vi "Save Image.vi"(8 "error in (no error)":errorcluster, 11 "Save Image in":refnum<class "Save Image.lvclass">) -> (0 "error out":errorcluster, 3 "Save Image out":refnum<class "Save Image.lvclass">)   [LabVIEW 2018, in "Save Image.lvclass"]
uses:
  Save Image.lvclass
  <userlib>/gfitsio/cfitsio-bitpix.ctl
  Save Image.lvclass/Save Image.ctl
  <userlib>/gfitsio/gfitsio-write-image-subset-variant.vi
  <userlib>/gfitsio/gfitsio.lvlib
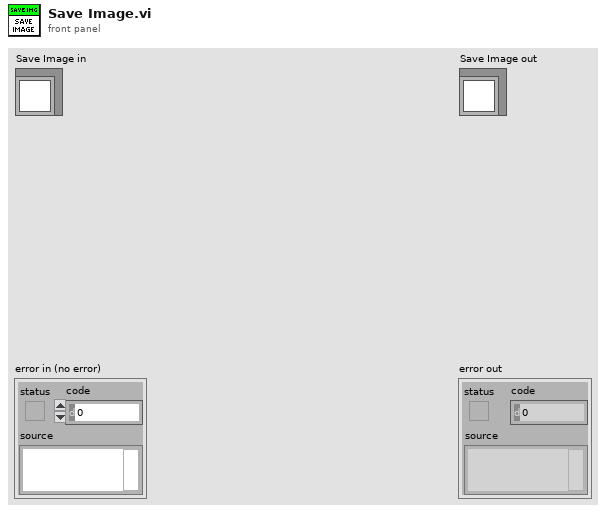
[diagram p1: front panel]
types:
  T1 = enum16{"open", "open or create", "create or replace", "create", "open (read only)"}
  T2 = enum16{"open", "open or create", "create", "create or replace"}
  T3 = typedef "gfitsio.lvlib/cfitsio-bitpix.ctl" = i32
  T4 = typedef "gfitsio.lvlib/gfitsio-refnum.ctl" = refnum<k1>
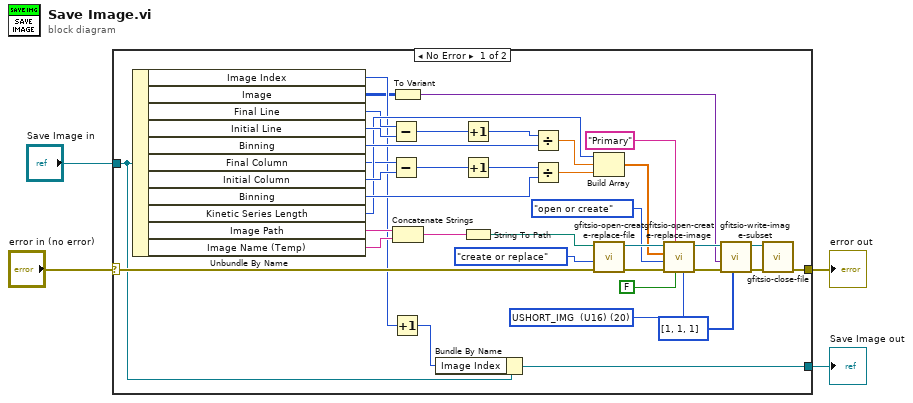
[diagram p0: block diagram]
diagram:
  n1 = case shown="No Error" "error in (no error)" {
    selector: "error in (no error)" -> [w21 w44]
    tunnel: [w42 w44] -> w2
    tunnel: "Save Image in" -> [w15 w43]
    tunnel: [w14 w43] -> w1
    frame No Error {
      w37 = T3 20 items=["<invalid type>"=0, "BYTE_IMG  (U8)"=8, "SHORT_IMG  (I16)"=16, "USHORT_IMG  (U16)"=20, "LONG_IMG  (I32)"=32, "ULONG_IMG  (U32)"=40, "FLOAT_IMG  (SGL)"=-32, "DOUBLE_IMG  (DBL)"=-64] ("image data type")
      n2 = Unbundle By Name(w15) -> ("Image Index"=w12:u16, "Image"=w5:u16[][][], "Final Line"=w18:u16, "Initial Line"=w29:u16, "Binning"=w30:u16, "Final Column"=w17:u16, "Initial Column"=w31:u16, "Binning"=w32:u16, "Kinetic Series Length"=w19:u16, "Image Path"=w16:string, "Image Name (Temp)"=w20:string)
      n3 = Subtract(x=w18, y=w29) -> (x-y=w27:u16)
      n4 = Subtract(x=w17, y=w31) -> (x-y=w28:u16)
      n5 = Increment(x=w12) -> (x+1=w13:u16)
      n6 = To Variant(anything=w5) -> (Variant=w6:variant)
      n7 = Concatenate Strings(w16, w20) -> (w36:string)
      n8 = Bundle By Name(cluster=w15, "Image Index"=w13) -> (w14:refnum<class "Save Image.lvclass">)
      n9 = Increment(x=w27) -> (x+1=w11:u16)
      n10 = Increment(x=w28) -> (x+1=w10:u16)
      n11 = String To Path(string=w36) -> (path=w35:path)
      n12 = Divide(x=w11, y=w30) -> (x/y=w9:dbl)
      n13 = Divide(x=w10, y=w32) -> (x/y=w8:dbl)
      n14 = Build Array(w19, w9, w8) -> (w26:dbl[])
      n15 = call <userlib>:"gfitsio-open-create-replace-file.vi"("error in (no error)"=w21, "function (open)"=T1."create or replace", "file path (dialog if empty)"=w35) -> ("error out"=w41:errorcluster, "gfits refnum"=w40:T4)  [unwired: 6 in, 1 out]
      n16 = call <userlib>:"gfitsio-open-create-replace-image.vi"("image data type"=w37, "advisory dialog? (display:T)"=FALSE, "hdu name (dialog if empty)"="Primary" ("prompt"), "error in (no error)"=w41, "function (create or replace)"=T2."open or create" ("function (open or create)"), "naxes"=w26, "gfits refnum"=w40) -> ("error out"=w22:errorcluster, "dup gfits refnum"=w23:T4)  [unwired: 2 in, 1 out]
      n17 = call-poly <userlib>:"gfitsio-write-image-subset.vi"("fpixel"=i32[] [1, 1, 1], "error in (no error)"=w22, "data"=w6, "gfits refnum"=w23) -> ("error out"=w25:errorcluster, "dup gfits refnum"=w24:T4)  [unwired: 6 in]
      n18 = call <userlib>:"gfitsio-close-file.vi"("error in (no error)"=w25, "gfits refnum"=w24) -> ("error out"=w42:errorcluster)  [unwired: 8 in, 1 out]
    }
    frame Error {
    }
  }
  "error out" <- w2
  "Save Image out" <- w1
